vi "Get DO param from PGserver.vi"(6 "conninfo":T1={"host"="localhost", "port"="5432", "client_encoding"="WIN1251", "dbname"="system", "user"="postgres", "password"=""}, 7 "KFM":string[](array[string]), 8 "error in (no error)":errorcluster, 9 "DOParamColumns":string[](array[string])=["module_fcode_full", "control_channel_num", "fcode_full", "fname"], 10 "DOParamTable":string="fdo_1", 11 "DO_fcode_full":string[](array[string])) -> (0 "error out":errorcluster, 2 "Names table":string[][](array[string]), 3 "DOParameters table":dbl[][](array[numeric]))   [LabVIEW 2019, in "Inputs.lvlib"]
uses:
  Inputs.lvlib
  Database/ctl/Coninfo.ctl
  Database/PostgreSQL2LabVIEW/libpqUtility64/src/PQfetchResultData.vi
  Database/PostgreSQL2LabVIEW/libpqlv64/src/PQresultErrorMessage.vi
  Database/PostgreSQL2LabVIEW/libpqlv64/src/PQresultStatus.vi
  Database/PostgreSQL2LabVIEW/libpqlv64/src/PQsendQuery.vi
  Database/PostgreSQL2LabVIEW/libpqlv64/src/PQgetResult.vi
  Database/PostgreSQL2LabVIEW/libpqUtility64/src/PQclear.vi
  Database/PostgreSQL2LabVIEW/libpqlv64/src/PQfinish.vi
  Database/PostgreSQL2LabVIEW/libpqlv64/src/PQconnectdb.vi
  Database/PostgreSQL2LabVIEW/libpqlv64/src/PQerrorMessage.vi
  Database/PostgreSQL2LabVIEW/libpqlv64/src/PQstatus.vi
  <vilib>/dlg_ctls.llb/Space Constant.vi
  Database/PostgreSQL2LabVIEW/libpqlv64/src/PQgetvalue.vi
  Database/PostgreSQL2LabVIEW/libpqlv64/src/PQnfields.vi
  Database/PostgreSQL2LabVIEW/libpqlv64/src/PQntuples.vi
  Database/PostgreSQL2LabVIEW/libpqlv64/src/PQclear.vi
  Database/Progress.vi
  Database/PostgreSQL.lvlib
  Database/PostgreSQL2LabVIEW/libpqUtility/libpqutility.lvlib
  Database/PostgreSQL2LabVIEW/libpqUtility64/libpqutility64.lvlib
panel:
  out "PQStatus":T2(ring)
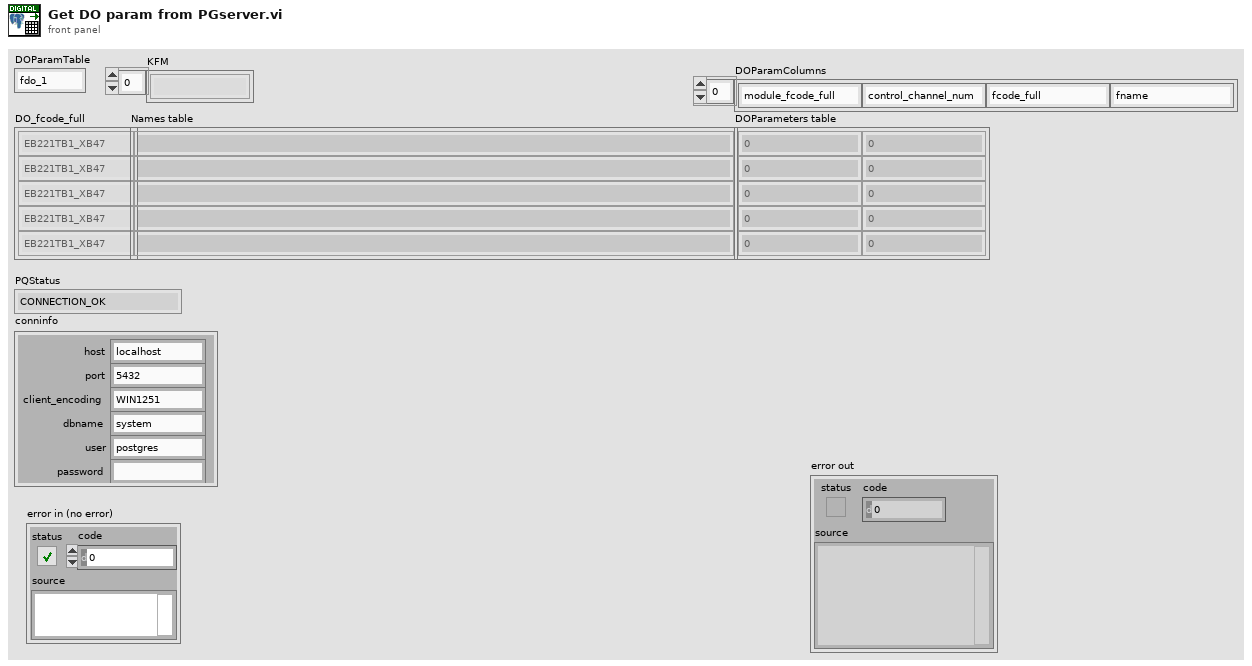
[diagram p1: front panel]
types:
  T1 = typedef "PostgreSQL.lvlib/Coninfo.ctl" = cluster{"host":string, "port":string, "client_encoding":string, "dbname":string, "user":string, "password":string}
  T2 = enum16{"CONNECTION_OK", "CONNECTION_BAD", "CONNECTION_STARTED", "CONNECTION_MADE", "CONNECTION_AWAITING_RESPONSE", "CONNECTION_AUTH_OK", "CONNECTION_SETENV", "CONNECTION_SSL_STARTUP", "CONNECTION_NEEDED"}
  T3 = enum32{"CONNECTION_OK", "CONNECTION_BAD", "CONNECTION_STARTED", "CONNECTION_MADE", "CONNECTION_AWAITING_RESPONSE", "CONNECTION_AUTH_OK", "CONNECTION_SETENV", "CONNECTION_SSL_STARTUP", "CONNECTION_NEEDED"}
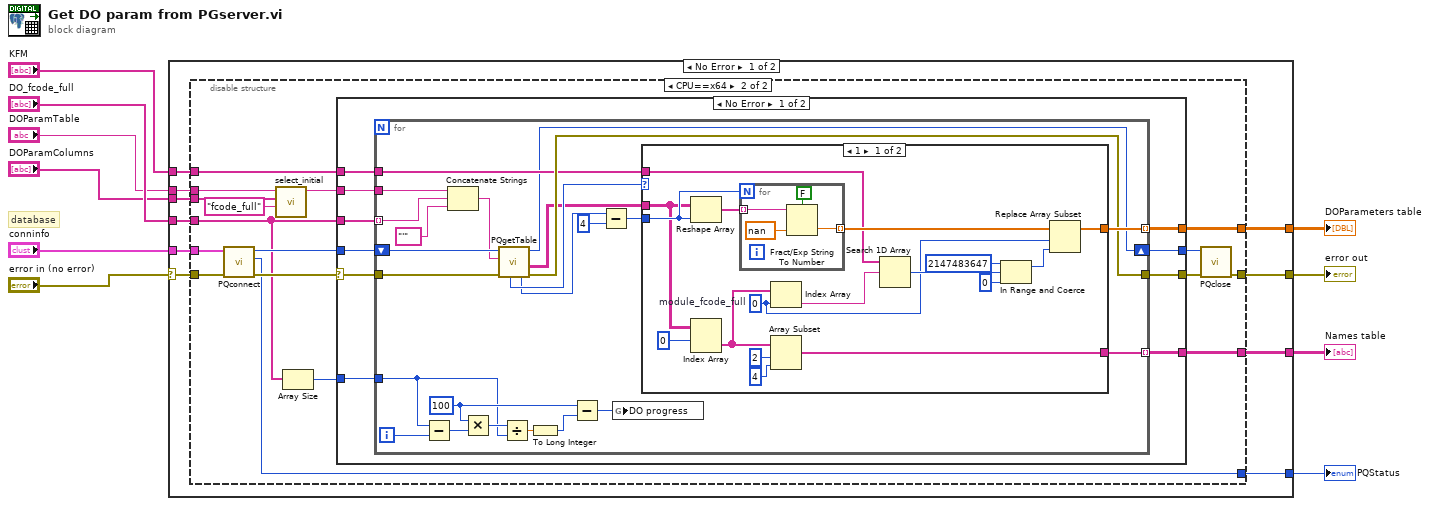
[diagram p0: block diagram]
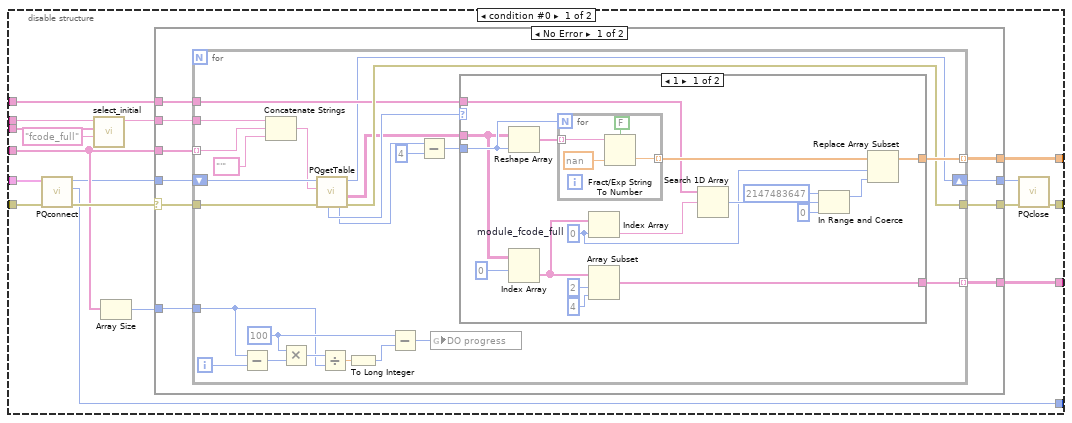
[diagram p2: hidden frame]
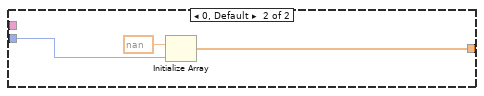
[diagram p3: hidden frame]
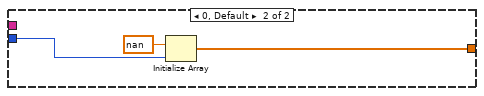
[diagram p5: hidden frame]
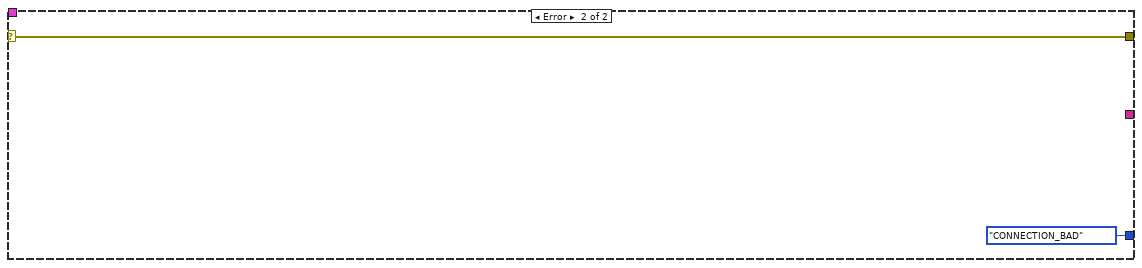
[diagram p7: hidden frame]
diagram:
  # "database"
  n1 = case shown="No Error" "error in (no error)" {
    selector: "error in (no error)" -> [w13 w176]
    tunnel: "DO_fcode_full" -> [w20 _]
    tunnel: "DOParamTable" -> [w18 _]
    tunnel: "DOParamColumns" -> [w17 _]
    tunnel: [w19 _] -> w7
    tunnel: [w16 w176] -> w6
    tunnel: [w15 _] -> w5
    tunnel: "conninfo" -> [w14 _]
    tunnel: "KFM" -> [w12 _]
    tunnel: [w11 T3."CONNECTION_BAD" ("PQStatus")] -> w1
    frame No Error {
      n2 = disable-structure shown="CPU==x64" {
        disable-tunnel: w20 -> [w36 w101]
        disable-tunnel: [w35 w107] -> w19
        disable-tunnel: w18 -> [w33 w99]
        disable-tunnel: w17 -> [w32 w100]
        disable-tunnel: [w31 w106] -> w16
        disable-tunnel: [w30 w105] -> w15
        disable-tunnel: w14 -> [w29 w102]
        disable-tunnel: w13 -> [w28 w103]
        disable-tunnel: w12 -> [w27 w98]
        disable-tunnel: [w23 w104] -> w11
        frame condition #0 {
          n3 = call "PQconnect.vi"("error in (no error)"=w28, "conninfo"=w29) -> ("error out"=w37:errorcluster, "PQStatus"=w23:T3, "conn"=w22:u32)  [unwired: 7 in]
          n4 = call "select_initial.vi"("Column name"="fcode_full", "Column table"=w32, "table"=w33) -> ("parameters"=w25:string)  [unwired: 7 in, 1 out]
          n5 = Array Size(array=w36) -> (size(s)=w26:i32)
          n6 = case shown="No Error" w37 {
            selector: w37 -> [w46 w97]
            tunnel: w36 -> [w44 _]
            tunnel: [w47 _] -> w35
            tunnel: [w41 _] -> w30
            tunnel: w26 -> [w45 _]
            tunnel: w22 -> [w43 w96]
            tunnel: w25 -> [w42 _]
            tunnel: [w40 w97] -> w34
            tunnel: w27 -> [w39 _]
            tunnel: [w38 w96] -> w21
            frame No Error {
              n7 = for {
                tunnel: [w71] -> w47 mode=indexing
                tunnel: w46 -> [w56]
                tunnel: w45 -> [w60]
                tunnel: w44 -> [w69] mode=indexing
                tunnel: w42 -> [w70]
                tunnel: [w58] -> w41 mode=indexing
                tunnel: [w54] -> w40
                tunnel: w39 -> [w51]
                shift-right: [w48] -> w38
                shift-left: w43 -> [w57]
                i -> [w61]
                w65 = 100 ("y")
                n8 = Subtract(x=w60, y=w61) -> (x-y=w64:i32)
                n9 = Concatenate Strings(w70, w69, "'" ("table")) -> (w55:string)
                n10 = Multiply(x=w65, y=w64) -> (x*y=w67:i32)
                n11 = call "PQgetTable.vi"("error in"=w56, "query"=w55, "conn"=w57) -> ("error out"=w54:errorcluster, "Data"=w52:string[][], "conn_out"=w48:u32, "PQnFields"=w50:i32, "PQnTuples"=w53:i32)  [unwired: 4 in]
                n12 = Divide(x=w67, y=w60) -> (x/y=w63:dbl)
                n13 = To Long Integer(number=w63) -> (32bit integer=w62:i32)
                n14 = Subtract(x=w65, y=w62) -> (x-y=w66:i32)
                n15 = Subtract(x=w50, y=u32 4) -> (x-y=w59:u32)
                n16 = global write "Progress.vi" "DO progress"(w66) -> ()
                n17 = case shown="1" w53 {
                  tunnel: [w77 w94] -> w71
                  tunnel: w59 -> [w87 w93]
                  tunnel: w52 -> [w86 _]
                  tunnel: [w82 _] -> w58
                  tunnel: w51 -> [w73 _]
                  frame 1 {
                    w72 = 0  # module_fcode_full
                    n18 = Reshape Array(w86, w87) -> (w88:string[])
                    n19 = Index Array(array=w86, index (row)=0 ("disabled index (row)")) -> (element=w74:string[])  [unwired: 1 in]
                    n20 = for {
                      N: w87 -> [_]
                      tunnel: w88 -> [w91] mode=indexing
                      tunnel: [w90] -> w76 mode=indexing
                      n21 = Fract/Exp String To Number(use system decimal point (T)=FALSE, string=w91, default (0 dbl)=nan) -> (number=w90:dbl)  [unwired: 1 in, 1 out]
                    }
                    n22 = Index Array(array=w74, index=w72) -> (element=w75:string)
                    n23 = Array Subset(array=w74, index=2, length=4) -> (w82:string[])
                    n24 = Search 1D Array(1D array=w73, element=w75) -> (index of element=w80:i32)  [unwired: 1 in]
                    n25 = In Range and Coerce(upper limit=2147483647, x=w80, lower limit=0) -> (coerced(x)=w78:i32)  [unwired: 1 out]
                    n26 = Replace Array Subset(array=w76, new element=w78, index=w72) -> (w77:dbl[])
                  }
                  frame 0, Default {
                    n27 = Initialize Array(nan, w93) -> (w94:dbl[])
                  }
                }
              }
            }
            frame Error {
            }
          }
          n28 = call "PQclose.vi"("error in (no error)"=w34, "conn"=w21) -> ("error out"=w31:errorcluster)  [unwired: 9 in]
        }
        frame condition #1 (active) {
          n29 = call "PQconnect.vi"("error in (no error)"=w103, "conninfo"=w102) -> ("error out"=w114:errorcluster, "PQStatus"=w104:T3, "conn"=w109:u64)  [unwired: 7 in]
          n30 = call "select_initial.vi"("Column name"="fcode_full", "Column table"=w100, "table"=w99) -> ("parameters"=w111:string)  [unwired: 7 in, 1 out]
          n31 = Array Size(array=w101) -> (size(s)=w112:i32)
          n32 = case shown="No Error" w114 {
            selector: w114 -> [w123 w174]
            tunnel: w101 -> [w121 _]
            tunnel: [w124 _] -> w107
            tunnel: [w118 _] -> w105
            tunnel: w112 -> [w122 _]
            tunnel: w109 -> [w120 w173]
            tunnel: w111 -> [w119 _]
            tunnel: [w117 w174] -> w113
            tunnel: w98 -> [w116 _]
            tunnel: [w115 w173] -> w108
            frame No Error {
              n33 = for {
                tunnel: [w148] -> w124 mode=indexing
                tunnel: w123 -> [w133]
                tunnel: w122 -> [w137]
                tunnel: w121 -> [w146] mode=indexing
                tunnel: w119 -> [w147]
                tunnel: [w135] -> w118 mode=indexing
                tunnel: [w131] -> w117
                tunnel: w116 -> [w128]
                shift-right: [w125] -> w115
                shift-left: w120 -> [w134]
                i -> [w138]
                w142 = 100 ("y")
                n34 = Subtract(x=w137, y=w138) -> (x-y=w141:i32)
                n35 = Concatenate Strings(w147, w146, "'" ("table")) -> (w132:string)
                n36 = Multiply(x=w142, y=w141) -> (x*y=w144:i32)
                n37 = call "PQgetTable.vi"("error in"=w133, "query"=w132, "conn"=w134) -> ("error out"=w131:errorcluster, "Data"=w129:string[][], "conn_out"=w125:u64, "PQnFields"=w127:i64, "PQnTuples"=w130:i64)  [unwired: 4 in]
                n38 = Divide(x=w144, y=w137) -> (x/y=w140:dbl)
                n39 = To Long Integer(number=w140) -> (32bit integer=w139:i32)
                n40 = Subtract(x=w142, y=w139) -> (x-y=w143:i32)
                n41 = Subtract(x=w127, y=i64 4) -> (x-y=w136:i64)
                n42 = global write "Progress.vi" "DO progress"(w143) -> ()
                n43 = case shown="1" w130 {
                  tunnel: [w154 w171] -> w148
                  tunnel: w136 -> [w164 w170]
                  tunnel: w129 -> [w163 _]
                  tunnel: [w159 _] -> w135
                  tunnel: w128 -> [w150 _]
                  frame 1 {
                    w149 = 0  # module_fcode_full
                    n44 = Reshape Array(w163, w164) -> (w165:string[])
                    n45 = Index Array(array=w163, index (row)=0 ("disabled index (row)")) -> (element=w151:string[])  [unwired: 1 in]
                    n46 = for {
                      N: w164 -> [_]
                      tunnel: w165 -> [w168] mode=indexing
                      tunnel: [w167] -> w153 mode=indexing
                      n47 = Fract/Exp String To Number(use system decimal point (T)=FALSE, string=w168, default (0 dbl)=nan) -> (number=w167:dbl)  [unwired: 1 in, 1 out]
                    }
                    n48 = Index Array(array=w151, index=w149) -> (element=w152:string)
                    n49 = Array Subset(array=w151, index=2, length=4) -> (w159:string[])
                    n50 = Search 1D Array(1D array=w150, element=w152) -> (index of element=w157:i32)  [unwired: 1 in]
                    n51 = In Range and Coerce(upper limit=2147483647, x=w157, lower limit=0) -> (coerced(x)=w155:i32)  [unwired: 1 out]
                    n52 = Replace Array Subset(array=w153, new element=w155, index=w149) -> (w154:dbl[])
                  }
                  frame 0, Default {
                    n53 = Initialize Array(nan, w170) -> (w171:dbl[])
                  }
                }
              }
            }
            frame Error {
            }
          }
          n54 = call "PQclose.vi"("error in (no error)"=w113, "conn"=w108) -> ("error out"=w106:errorcluster)  [unwired: 9 in]
        }
      }
    }
    frame Error {
    }
  }
  "error out" <- w6
  "DOParameters table" <- w7
  "Names table" <- w5
  "PQStatus" <- w1
